vi "ErrorStateLogger.vi"(10 "error in":errorcluster, 11 "String":string) -> ()   [LabVIEW 2019]
panel:
  out "Array":T1(array[cluster])
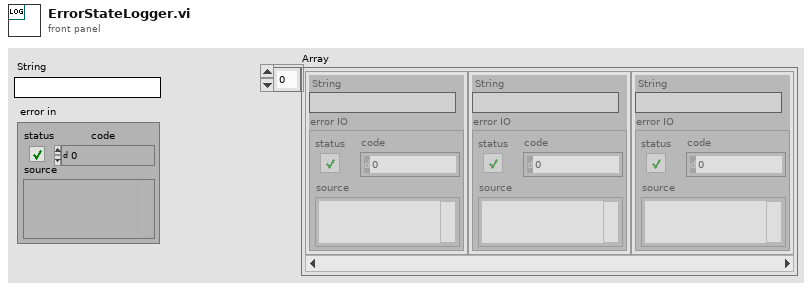
[diagram p1: front panel]
types:
  T1 = cluster{"String":string, "error IO":errorcluster}[]
  T2 = cluster{"String":string, "error IO":errorcluster}
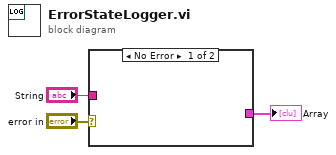
[diagram p0: block diagram]
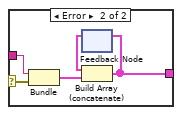
[diagram p2: hidden frame]
diagram:
  n1 = case shown="No Error" "error in" {
    selector: "error in" -> [_ w7]
    tunnel: "String" -> [_ w6]
    tunnel: [_ w4] -> w1
    frame No Error {
    }
    frame Error {
      n2 = Bundle("String"=w6, "error IO"=w7) -> (w5:T2)  [unwired: 1 in]
      n3 = feedback #1() -> (w8:T1)  [unwired: 1 in]
      n4 = Build Array (concatenate)(w8, w5) -> (w4:T1)
      n5 = feedback-in #1(w4) -> ()
    }
  }
  "Array" <- w1
